vi "Destroy User Events_RC.vi"(8 "error in (no error)":errorcluster, 11 "Rack Controller in":refnum<class "Rack Controller.lvclass">) -> (0 "error out":errorcluster)   [LabVIEW 2019, in "Rack Controller.lvclass"]
uses:
  Rack Controller.lvclass
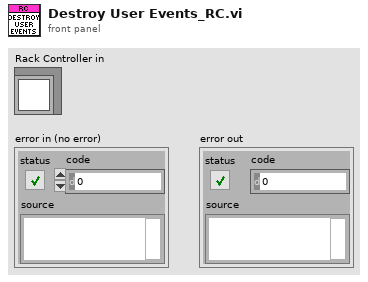
[diagram p1: front panel]
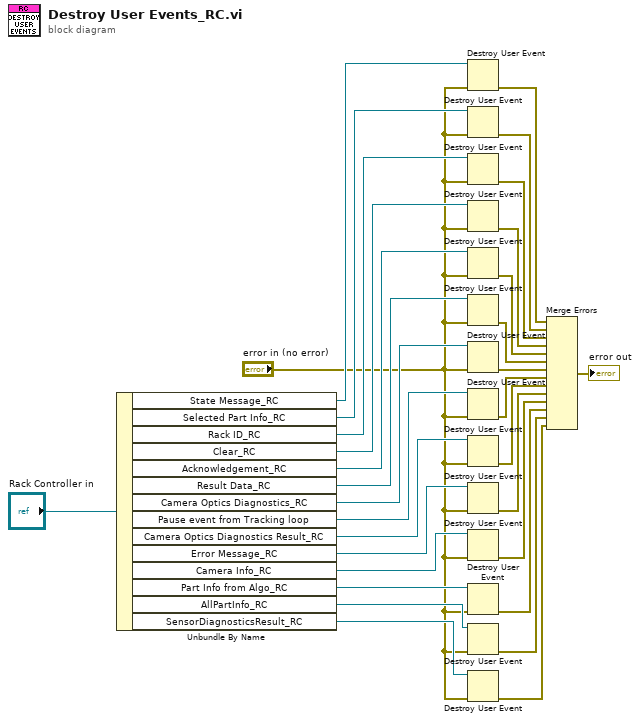
[diagram p0: block diagram]
diagram:
  n1 = Unbundle By Name("Rack Controller in") -> ("State Message_RC"=w28:refnum<user-event>, "Selected Part Info_RC"=w29:refnum<user-event>, "Rack ID_RC"=w30:refnum<user-event>, "Clear_RC"=w16:refnum<user-event>, "Acknowledgement_RC"=w15:refnum<user-event>, "Result Data_RC"=w14:refnum<user-event>, "Camera Optics Diagnostics_RC"=w13:refnum<user-event>, "Pause event from Tracking loop"=w12:refnum<user-event>, "Camera Optics Diagnostics Result_RC"=w11:refnum<user-event>, "Error Message_RC"=w10:refnum<user-event>, "Camera Info_RC"=w9:refnum<user-event>, "Part Info from Algo_RC"=w8:refnum<user-event>, "AllPartInfo_RC"=w7:refnum<user-event>, "SensorDiagnosticsResult_RC"=w6:refnum<user-event>)
  n2 = Destroy User Event(user event=w28, error in="error in (no error)") -> (error out=w27:errorcluster)
  n3 = Destroy User Event(user event=w29, error in="error in (no error)") -> (error out=w26:errorcluster)
  n4 = Destroy User Event(user event=w30, error in="error in (no error)") -> (error out=w25:errorcluster)
  n5 = Destroy User Event(user event=w16, error in="error in (no error)") -> (error out=w24:errorcluster)
  n6 = Destroy User Event(user event=w15, error in="error in (no error)") -> (error out=w23:errorcluster)
  n7 = Destroy User Event(user event=w14, error in="error in (no error)") -> (error out=w22:errorcluster)
  n8 = Destroy User Event(user event=w13, error in="error in (no error)") -> (error out=w21:errorcluster)
  n9 = Destroy User Event(user event=w12, error in="error in (no error)") -> (error out=w20:errorcluster)
  n10 = Destroy User Event(user event=w11, error in="error in (no error)") -> (error out=w19:errorcluster)
  n11 = Destroy User Event(user event=w10, error in="error in (no error)") -> (error out=w18:errorcluster)
  n12 = Destroy User Event(user event=w9, error in="error in (no error)") -> (error out=w4:errorcluster)
  n13 = Destroy User Event(user event=w8, error in="error in (no error)") -> (error out=w3:errorcluster)
  n14 = Destroy User Event(user event=w7, error in="error in (no error)") -> (error out=w2:errorcluster)
  n15 = Destroy User Event(user event=w6, error in="error in (no error)") -> (error out=w1:errorcluster)
  n16 = Merge Errors(w27, w26, w25, w24, w23, w22, w21, w20, w19, w18, w4, w3, w2, w1) -> (→"error out":errorcluster)
